vi "Automatic CE-CERT Inverter MODBUS TCP-IP Curtailment v2.vi"() -> ()   [LabVIEW 2018]
uses:
  <vilib>/Plasmionique/MB Master/MB_Master_TCP/MB_Master_TCP.lvclass
  C:/Program Files (x86)/National Instruments/LabVIEW 2018/vi.lib/Plasmionique/MB Master/MB_Master/MB_Master.lvclass
  <vilib>/Plasmionique/MB Master/MB Master.lvlib
panel:
  out "Current State Curtailment":T1(ring)
  in  "Curtailment Setpoint (%)":u16
  in  "Curtailment":bool
  in  "Power Factor":bool
  out "Inverter ready for commands?":bool
  in  "Power Factor Setpoint":i16
  out "Curtailment mode (should be 0 while not curtailing)":u16
  out "Power Factor Mode (should be 0 while not changing power factor)":u16
  out "Power Factor Operation Error (Should be 0)":u16
  out "Power Factor Format Error (Should be 0)":u16
  out "Current State Power Factor":T2(ring)
  in  "stop":bool
  in  "IP Address":string
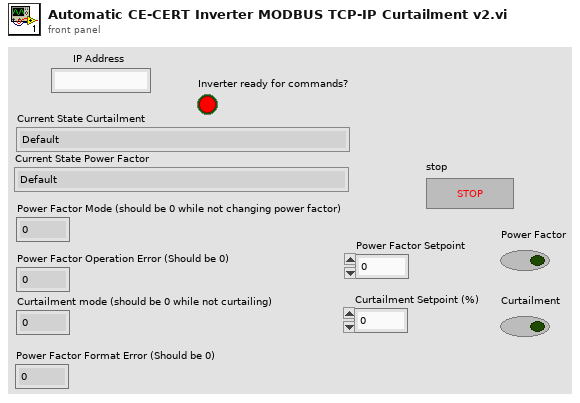
[diagram p1: front panel]
types:
  T1 = enum16{"Default", "Set advanced power control", "Set power factor mode", "set curtailment mode", "set ramp rate", "set action delay", "set randomize range", "set curtailment setpoint", "set go now command"}
  T2 = enum16{"Default", "Set Advanced power controls", "Set power factor mode", "set curtailment mode", "set action delay", "set ramp rate", "set randomize range", "set power factor setpoint", "set go now command"}
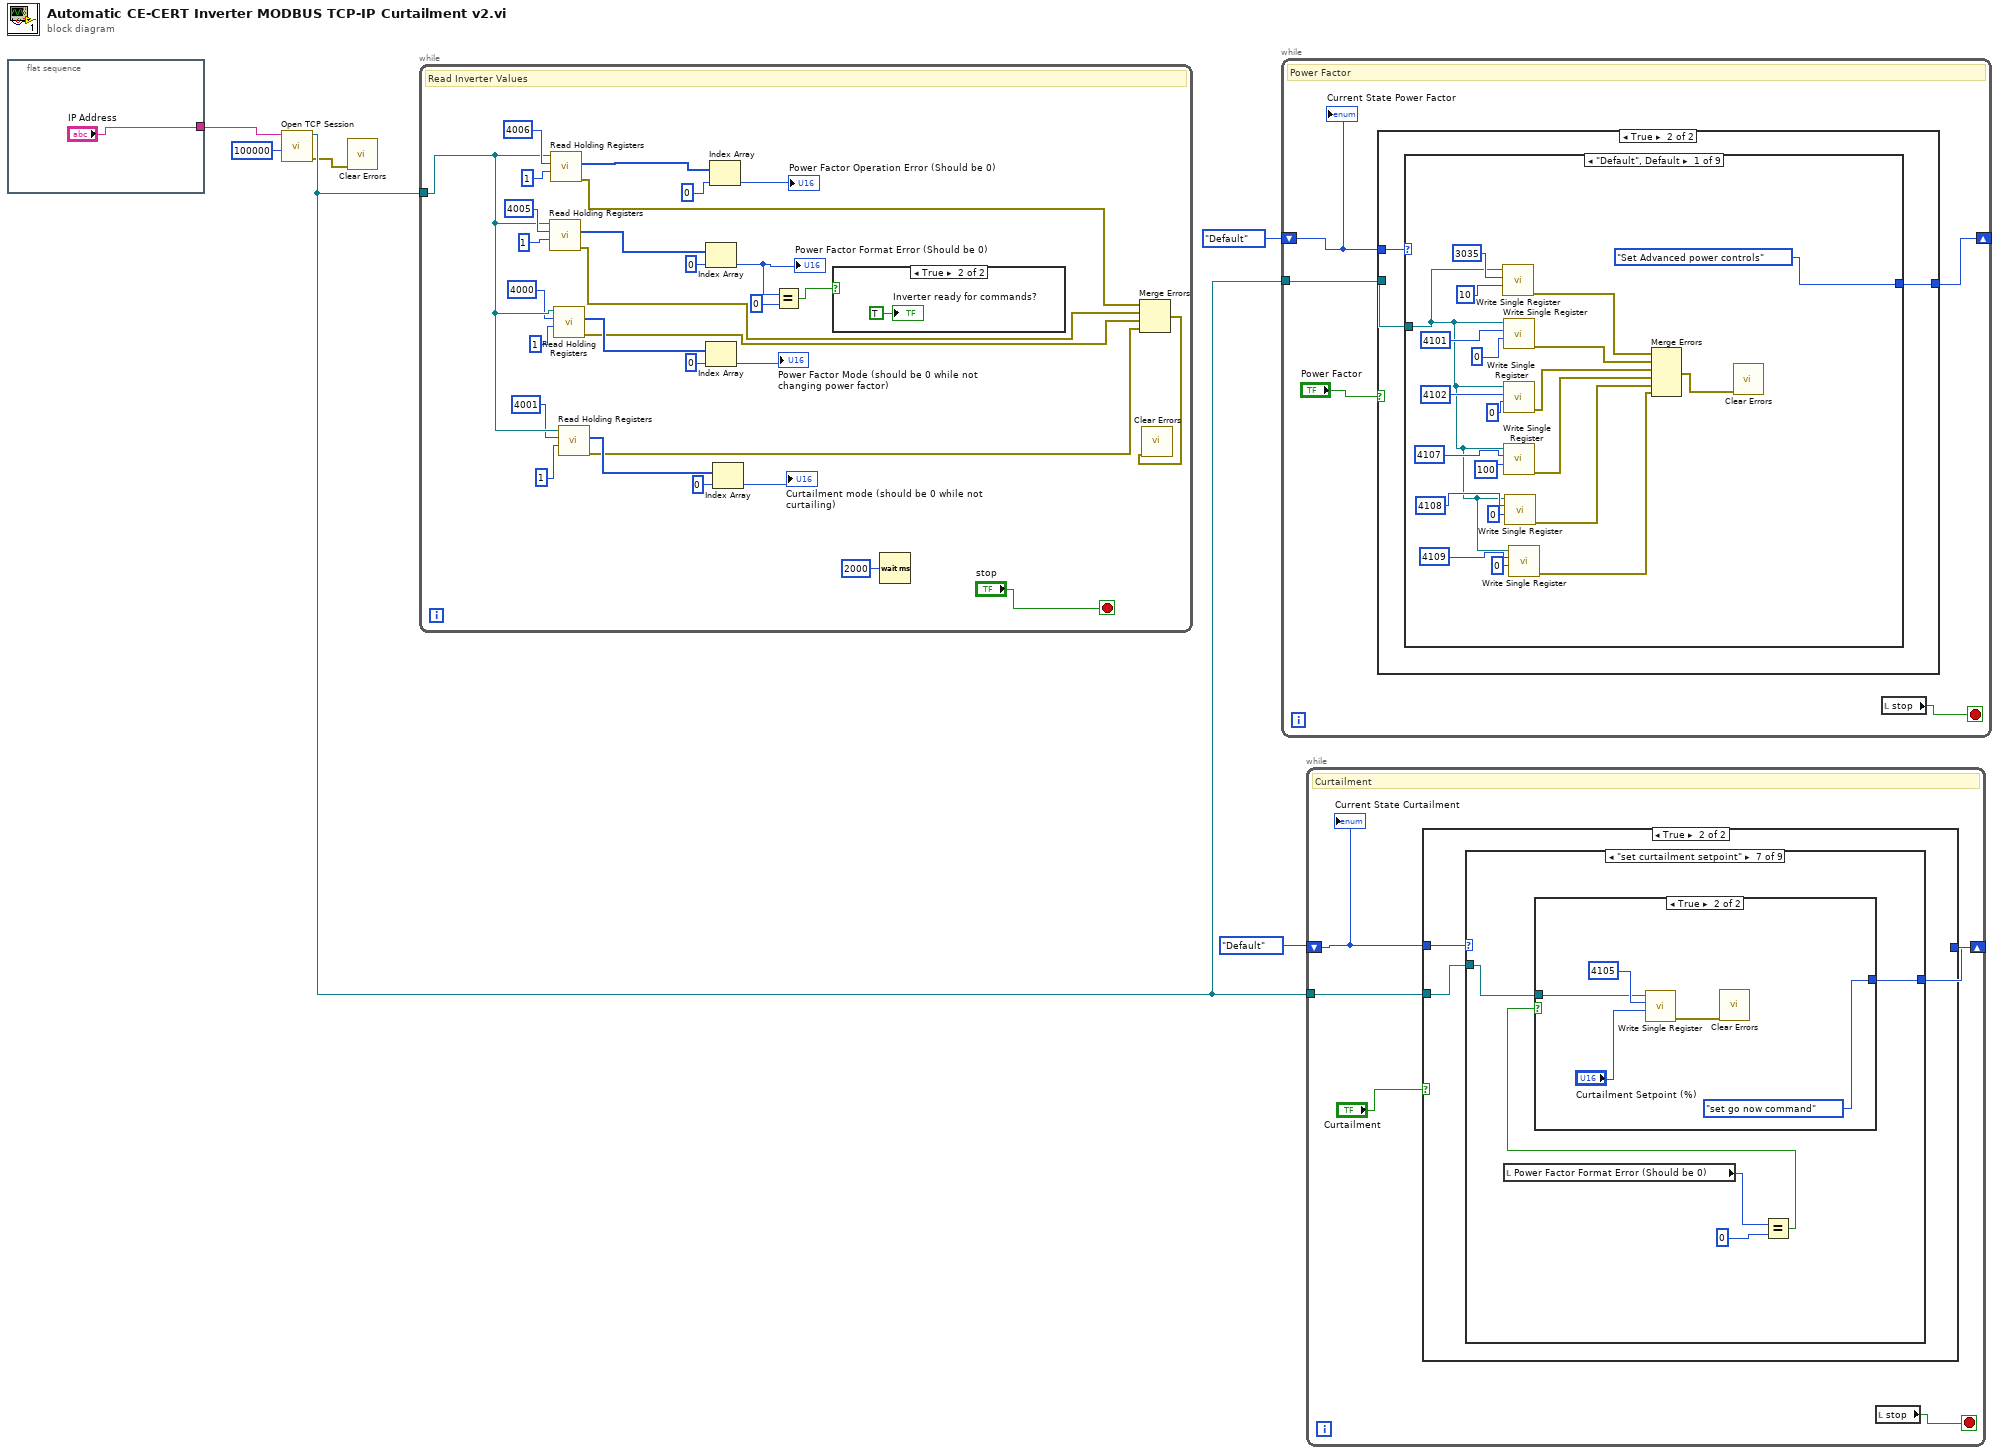
[diagram p0: block diagram]
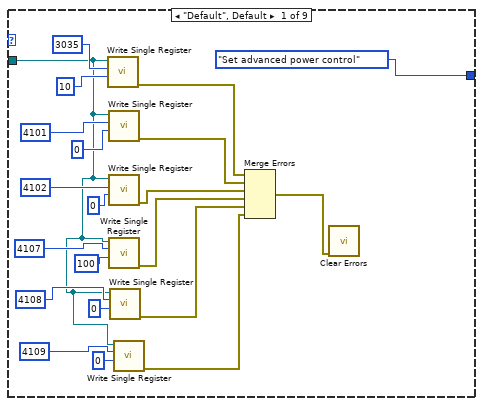
[diagram p3: hidden frame]
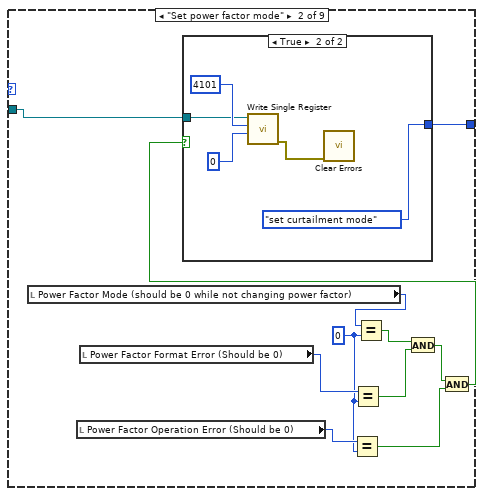
[diagram p4: hidden frame]
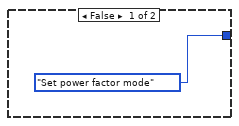
[diagram p5: hidden frame]
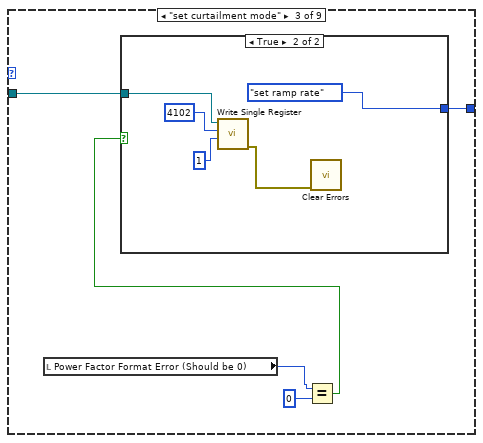
[diagram p6: hidden frame]
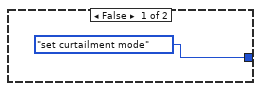
[diagram p7: hidden frame]
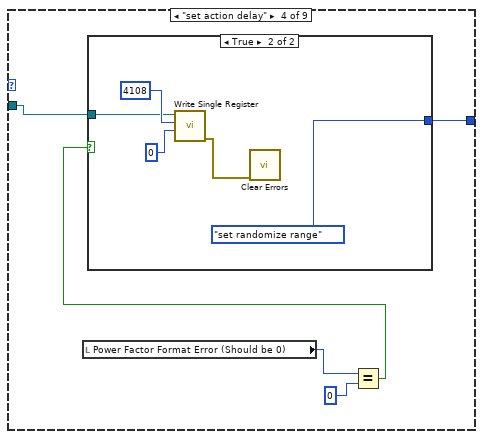
[diagram p8: hidden frame]
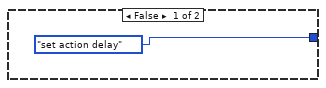
[diagram p9: hidden frame]
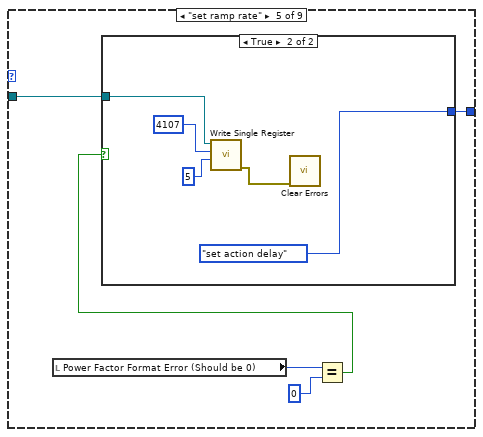
[diagram p10: hidden frame]
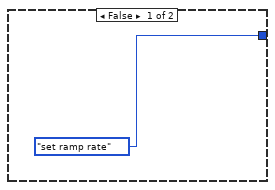
[diagram p11: hidden frame]
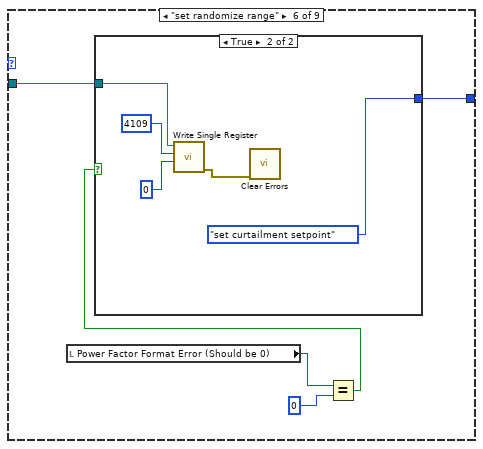
[diagram p12: hidden frame]
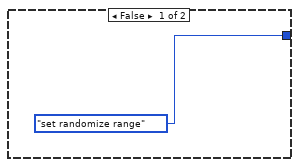
[diagram p13: hidden frame]
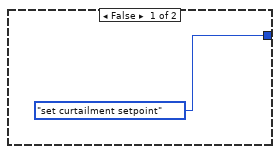
[diagram p14: hidden frame]
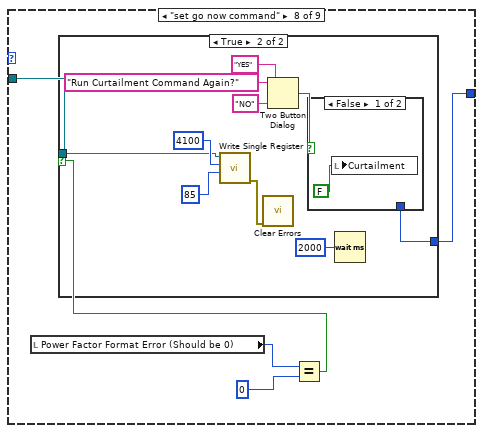
[diagram p15: hidden frame]
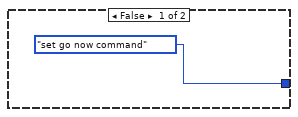
[diagram p16: hidden frame]
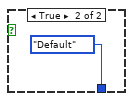
[diagram p17: hidden frame]
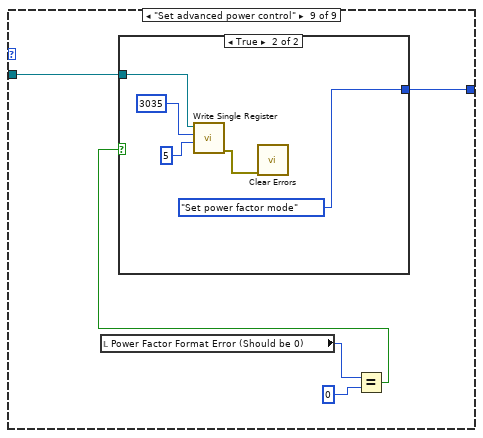
[diagram p18: hidden frame]
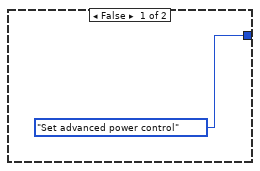
[diagram p19: hidden frame]
diagram:
  n1 = flat-sequence {
    tunnel: ["IP Address"] -> w6
    frame #0 {
    }
  }
  n2 = call <vilib>:"Open TCP Session.vi"("Timeout (10000)"=100000, "IP Address"=w6) -> ("error out"=w1:errorcluster, "MB_TCP session"=w3:refnum<class "MB_Master_TCP.lvclass">)  [unwired: 8 in]
  n3 = call <vilib>:"Clear Errors.vi"("error in (no error)"=w1) -> ()  [unwired: 5 in, 2 out]
  n4 = while {
    tunnel: w3 -> [w33]
    stop <- "stop" stop-if-true
    # "Read Inverter Values"
    n5 = call <vilib>:"Read Holding Registers.vi"("quantity"=u16 1, "starting address"=u16 4005, "MB session in"=w33) -> ("error out"=w11:errorcluster, "Registers"=w27:u16[])  [unwired: 6 in, 1 out]
    n6 = call <vilib>:"Read Holding Registers.vi"("quantity"=u16 1, "starting address"=u16 4006, "MB session in"=w33) -> ("error out"=w12:errorcluster, "Registers"=w25:u16[])  [unwired: 6 in, 1 out]
    n7 = call <vilib>:"Read Holding Registers.vi"("quantity"=u16 1, "starting address"=u16 4000, "MB session in"=w33) -> ("error out"=w10:errorcluster, "Registers"=w22:u16[])  [unwired: 6 in, 1 out]
    n8 = call <vilib>:"Read Holding Registers.vi"("quantity"=u16 1, "starting address"=u16 4001, "MB session in"=w33) -> ("error out"=w9:errorcluster, "Registers"=w19:u16[])  [unwired: 6 in, 1 out]
    n9 = Index Array(array=w27, index=0) -> (element=w16:u16)
    "Power Factor Format Error (Should be 0)" <- w16
    n10 = Index Array(array=w22, index=0) -> (element=→"Power Factor Mode (should be 0 while not changing power factor)":u16)
    n11 = Index Array(array=w25, index=0) -> (element=→"Power Factor Operation Error (Should be 0)":u16)
    n12 = Index Array(array=w19, index=0) -> (element=→"Curtailment mode (should be 0 while not curtailing)":u16)
    n13 = Equal?(x=w16, y=u16 0) -> (x = y?=w14:bool)
    n14 = case shown="True" w14 {
      frame False {
        n15 = local write "Inverter ready for commands?"(FALSE ("Inverter ready for commands")) -> ()
      }
      frame True {
        "Inverter ready for commands?" <- TRUE ("Inverter ready for commands")
      }
    }
    n16 = Wait (ms)(milliseconds to wait=u32 2000) -> ()  [unwired: 1 out]
    n17 = Merge Errors(w12, w11, w10, w9) -> (w8:errorcluster)
    n18 = call <vilib>:"Clear Errors.vi"("error in (no error)"=w8) -> ()  [unwired: 5 in, 2 out]
  }
  n19 = while {
    shift-right: [w41] -> _
    shift-left: T2."Default" -> [w43]
    tunnel: w3 -> [w42]
    stop <- w44 stop-if-true
    # "Power Factor"
    n20 = case shown="True" "Power Factor" {
      tunnel: w43 -> [_ w47]
      tunnel: w42 -> [_ w46]
      tunnel: [_ w45] -> w41
      frame False {
      }
      frame True {
        n21 = case shown="\"Default\", Default" w47 {
          tunnel: w46 -> [w56 w70 w87 w101 w109 w120 w131 w142 w160]
          tunnel: [T2."Set Advanced power controls" w69 w86 w97 w108 w119 w130 w141 w159] -> w45
          frame "Default", Default {
            n22 = call <vilib>:"Write Single Register.vi"("value"=u16 10, "address"=u16 3035, "MB session in"=w56) -> ("error out"=w54:errorcluster)  [unwired: 7 in, 1 out]
            n23 = call <vilib>:"Write Single Register.vi"("value"=u16 0, "address"=u16 4101, "MB session in"=w56) -> ("error out"=w53:errorcluster)  [unwired: 7 in, 1 out]
            n24 = call <vilib>:"Write Single Register.vi"("value"=u16 0, "address"=u16 4102, "MB session in"=w56) -> ("error out"=w52:errorcluster)  [unwired: 7 in, 1 out]
            n25 = call <vilib>:"Write Single Register.vi"("value"=u16 100, "address"=u16 4107, "MB session in"=w56) -> ("error out"=w51:errorcluster)  [unwired: 7 in, 1 out]
            n26 = call <vilib>:"Write Single Register.vi"("value"=u16 0, "address"=u16 4108, "MB session in"=w56) -> ("error out"=w50:errorcluster)  [unwired: 7 in, 1 out]
            n27 = call <vilib>:"Write Single Register.vi"("value"=u16 0, "address"=u16 4109, "MB session in"=w56) -> ("error out"=w49:errorcluster)  [unwired: 7 in, 1 out]
            n28 = Merge Errors(w54, w53, w52, w51, w50, w49) -> (w48:errorcluster)
            n29 = call <vilib>:"Clear Errors.vi"("error in (no error)"=w48) -> ()  [unwired: 5 in, 2 out]
          }
          frame "Set power factor mode" {
            w76 = u16 0 ("y")
            n30 = local read "Power Factor Mode (should be 0 while not changing power factor)"() -> (w79:u16)
            n31 = local read "Power Factor Operation Error (Should be 0)"() -> (w77:u16)
            n32 = local read "Power Factor Format Error (Should be 0)"() -> (w78:u16)
            n33 = Equal?(x=w77, y=w76) -> (x = y?=w72:bool)
            n34 = Equal?(x=w78, y=w76) -> (x = y?=w74:bool)
            n35 = Equal?(x=w79, y=w76) -> (x = y?=w75:bool)
            n36 = And(x=w75, y=w74) -> (x .and. y?=w73:bool)
            n37 = And(x=w73, y=w72) -> (x .and. y?=w71:bool)
            n38 = case shown="True" w71 {
              tunnel: w70 -> [_ w85]
              tunnel: [T2."Set power factor mode" T2."set curtailment mode"] -> w69
              frame False {
              }
              frame True {
                n39 = call <vilib>:"Write Single Register.vi"("value"=u16 1, "address"=u16 4101, "MB session in"=w85) -> ("error out"=w81:errorcluster)  [unwired: 7 in, 1 out]
                n40 = call <vilib>:"Clear Errors.vi"("error in (no error)"=w81) -> ()  [unwired: 5 in, 2 out]
              }
            }
          }
          frame "set curtailment mode" {
            n41 = local read "Power Factor Format Error (Should be 0)"() -> (w90:u16)
            n42 = Equal?(x=w90, y=u16 0) -> (x = y?=w88:bool)
            n43 = case shown="True" w88 {
              tunnel: w87 -> [_ w96]
              tunnel: [T2."set curtailment mode" T2."set action delay"] -> w86
              frame False {
              }
              frame True {
                n44 = call <vilib>:"Write Single Register.vi"("value"=u16 0, "address"=u16 4102, "MB session in"=w96) -> ("error out"=w92:errorcluster)  [unwired: 7 in, 1 out]
                n45 = call <vilib>:"Clear Errors.vi"("error in (no error)"=w92) -> ()  [unwired: 5 in, 2 out]
              }
            }
          }
          frame "set action delay" {
            n46 = local read "Power Factor Format Error (Should be 0)"() -> (w100:u16)
            n47 = Equal?(x=w100, y=u16 0) -> (x = y?=w98:bool)
            n48 = case shown="True" w98 {
              tunnel: w101 -> [_ w107]
              tunnel: [T2."set action delay" T2."set ramp rate"] -> w97
              frame False {
              }
              frame True {
                n49 = call <vilib>:"Write Single Register.vi"("value"=u16 0, "address"=u16 4108, "MB session in"=w107) -> ("error out"=w103:errorcluster)  [unwired: 7 in, 1 out]
                n50 = call <vilib>:"Clear Errors.vi"("error in (no error)"=w103) -> ()  [unwired: 5 in, 2 out]
              }
            }
          }
          frame "set ramp rate" {
            n51 = local read "Power Factor Format Error (Should be 0)"() -> (w111:u16)
            n52 = Equal?(x=w111, y=u16 0) -> (x = y?=w112:bool)
            n53 = case shown="True" w112 {
              tunnel: w109 -> [_ w118]
              tunnel: [T2."set ramp rate" T2."set randomize range"] -> w108
              frame False {
              }
              frame True {
                n54 = call <vilib>:"Write Single Register.vi"("value"=u16 100, "address"=u16 4107, "MB session in"=w118) -> ("error out"=w114:errorcluster)  [unwired: 7 in, 1 out]
                n55 = call <vilib>:"Clear Errors.vi"("error in (no error)"=w114) -> ()  [unwired: 5 in, 2 out]
              }
            }
          }
          frame "set randomize range" {
            n56 = local read "Power Factor Format Error (Should be 0)"() -> (w123:u16)
            n57 = Equal?(x=w123, y=u16 0) -> (x = y?=w121:bool)
            n58 = case shown="True" w121 {
              tunnel: w120 -> [_ w129]
              tunnel: [T2."set randomize range" T2."set power factor setpoint"] -> w119
              frame False {
              }
              frame True {
                n59 = call <vilib>:"Write Single Register.vi"("value"=u16 0, "address"=u16 4109, "MB session in"=w129) -> ("error out"=w125:errorcluster)  [unwired: 7 in, 1 out]
                n60 = call <vilib>:"Clear Errors.vi"("error in (no error)"=w125) -> ()  [unwired: 5 in, 2 out]
              }
            }
          }
          frame "set power factor setpoint" {
            n61 = local read "Power Factor Format Error (Should be 0)"() -> (w134:u16)
            n62 = Equal?(x=w134, y=u16 0) -> (x = y?=w132:bool)
            n63 = case shown="True" w132 {
              tunnel: w131 -> [_ w140]
              tunnel: [T2."set power factor setpoint" T2."set go now command"] -> w130
              frame False {
              }
              frame True {
                n64 = call <vilib>:"Write Single Register.vi"("value"="Power Factor Setpoint", "address"=u16 4103, "MB session in"=w140) -> ("error out"=w136:errorcluster)  [unwired: 7 in, 1 out]
                n65 = call <vilib>:"Clear Errors.vi"("error in (no error)"=w136) -> ()  [unwired: 5 in, 2 out]
              }
            }
          }
          frame "set go now command" {
            n66 = local read "Power Factor Format Error (Should be 0)"() -> (w145:u16)
            n67 = Equal?(x=w145, y=u16 0) -> (x = y?=w143:bool)
            n68 = case shown="True" w143 {
              tunnel: w142 -> [_ w156]
              tunnel: [T2."set go now command" w153] -> w141
              frame False {
              }
              frame True {
                n69 = call <vilib>:"Write Single Register.vi"("value"=u16 85, "address"=u16 4100, "MB session in"=w156) -> ("error out"=w147:errorcluster)  [unwired: 7 in, 1 out]
                n70 = Two Button Dialog(message="Run Power Factor Command again?", 1:"NO" ("T button name (\"OK\")"), 2:"YES" ("T button name (\"OK\")")) -> (T button?=w151:bool)
                n71 = call <vilib>:"Clear Errors.vi"("error in (no error)"=w147) -> ()  [unwired: 5 in, 2 out]
                n72 = case shown="True" w151 {
                  tunnel: [_ T2."Default"] -> w153
                  frame False {
                    n73 = local write "Power Factor"(FALSE ("Power Factor")) -> ()
                  }
                  frame True {
                  }
                }
                n74 = Wait (ms)(milliseconds to wait=u32 2000) -> ()  [unwired: 1 out]
              }
            }
          }
          frame "Set Advanced power controls" {
            n75 = local read "Power Factor Format Error (Should be 0)"() -> (w163:u16)
            n76 = Equal?(x=w163, y=u16 0) -> (x = y?=w161:bool)
            n77 = case shown="True" w161 {
              tunnel: w160 -> [_ w169]
              tunnel: [T2."Set Advanced power controls" T2."Set power factor mode"] -> w159
              frame False {
              }
              frame True {
                n78 = call <vilib>:"Write Single Register.vi"("value"=u16 5, "address"=u16 3035, "MB session in"=w169) -> ("error out"=w165:errorcluster)  [unwired: 7 in, 1 out]
                n79 = call <vilib>:"Clear Errors.vi"("error in (no error)"=w165) -> ()  [unwired: 5 in, 2 out]
              }
            }
          }
        }
      }
    }
    n80 = local read "stop"() -> (w44:bool)
    "Current State Power Factor" <- w43
  }
  n81 = while {
    tunnel: w3 -> [w173]
    shift-right: [w172] -> _
    shift-left: T1."Default" -> [w171]
    stop <- w174 stop-if-true
    # "Curtailment"
    n82 = case shown="True" "Curtailment" {
      tunnel: w173 -> [_ w177]
      tunnel: [_ w176] -> w172
      tunnel: w171 -> [_ w175]
      frame False {
      }
      frame True {
        n83 = case shown="\"set curtailment setpoint\"" w175 {
          tunnel: w177 -> [w186 w199 w216 w227 w238 w249 w260 w271 w289]
          tunnel: [T1."Set advanced power control" w200 w217 w228 w239 w250 w261 w272 w290] -> w176
          frame "Default", Default {
            n84 = call <vilib>:"Write Single Register.vi"("value"=u16 10, "address"=u16 3035, "MB session in"=w186) -> ("error out"=w184:errorcluster)  [unwired: 7 in, 1 out]
            n85 = call <vilib>:"Write Single Register.vi"("value"=u16 0, "address"=u16 4101, "MB session in"=w186) -> ("error out"=w183:errorcluster)  [unwired: 7 in, 1 out]
            n86 = call <vilib>:"Write Single Register.vi"("value"=u16 0, "address"=u16 4102, "MB session in"=w186) -> ("error out"=w182:errorcluster)  [unwired: 7 in, 1 out]
            n87 = call <vilib>:"Write Single Register.vi"("value"=u16 100, "address"=u16 4107, "MB session in"=w186) -> ("error out"=w181:errorcluster)  [unwired: 7 in, 1 out]
            n88 = call <vilib>:"Write Single Register.vi"("value"=u16 0, "address"=u16 4108, "MB session in"=w186) -> ("error out"=w180:errorcluster)  [unwired: 7 in, 1 out]
            n89 = call <vilib>:"Write Single Register.vi"("value"=u16 0, "address"=u16 4109, "MB session in"=w186) -> ("error out"=w179:errorcluster)  [unwired: 7 in, 1 out]
            n90 = Merge Errors(w184, w183, w182, w181, w180, w179) -> (w178:errorcluster)
            n91 = call <vilib>:"Clear Errors.vi"("error in (no error)"=w178) -> ()  [unwired: 5 in, 2 out]
          }
          frame "Set power factor mode" {
            w206 = u16 0 ("y")
            n92 = local read "Power Factor Mode (should be 0 while not changing power factor)"() -> (w209:u16)
            n93 = local read "Power Factor Operation Error (Should be 0)"() -> (w207:u16)
            n94 = local read "Power Factor Format Error (Should be 0)"() -> (w208:u16)
            n95 = Equal?(x=w207, y=w206) -> (x = y?=w202:bool)
            n96 = Equal?(x=w208, y=w206) -> (x = y?=w204:bool)
            n97 = Equal?(x=w209, y=w206) -> (x = y?=w205:bool)
            n98 = And(x=w205, y=w204) -> (x .and. y?=w203:bool)
            n99 = And(x=w203, y=w202) -> (x .and. y?=w201:bool)
            n100 = case shown="True" w201 {
              tunnel: [T1."Set power factor mode" T1."set curtailment mode"] -> w200
              tunnel: w199 -> [_ w212]
              frame False {
              }
              frame True {
                n101 = call <vilib>:"Write Single Register.vi"("value"=u16 0, "address"=u16 4101, "MB session in"=w212) -> ("error out"=w211:errorcluster)  [unwired: 7 in, 1 out]
                n102 = call <vilib>:"Clear Errors.vi"("error in (no error)"=w211) -> ()  [unwired: 5 in, 2 out]
              }
            }
          }
          frame "set curtailment mode" {
            n103 = local read "Power Factor Format Error (Should be 0)"() -> (w220:u16)
            n104 = Equal?(x=w220, y=u16 0) -> (x = y?=w218:bool)
            n105 = case shown="True" w218 {
              tunnel: [T1."set curtailment mode" T1."set ramp rate"] -> w217
              tunnel: w216 -> [_ w223]
              frame False {
              }
              frame True {
                n106 = call <vilib>:"Write Single Register.vi"("value"=u16 1, "address"=u16 4102, "MB session in"=w223) -> ("error out"=w222:errorcluster)  [unwired: 7 in, 1 out]
                n107 = call <vilib>:"Clear Errors.vi"("error in (no error)"=w222) -> ()  [unwired: 5 in, 2 out]
              }
            }
          }
          frame "set action delay" {
            n108 = local read "Power Factor Format Error (Should be 0)"() -> (w231:u16)
            n109 = Equal?(x=w231, y=u16 0) -> (x = y?=w229:bool)
            n110 = case shown="True" w229 {
              tunnel: [T1."set action delay" T1."set randomize range"] -> w228
              tunnel: w227 -> [_ w234]
              frame False {
              }
              frame True {
                n111 = call <vilib>:"Write Single Register.vi"("value"=u16 0, "address"=u16 4108, "MB session in"=w234) -> ("error out"=w233:errorcluster)  [unwired: 7 in, 1 out]
                n112 = call <vilib>:"Clear Errors.vi"("error in (no error)"=w233) -> ()  [unwired: 5 in, 2 out]
              }
            }
          }
          frame "set ramp rate" {
            n113 = local read "Power Factor Format Error (Should be 0)"() -> (w241:u16)
            n114 = Equal?(x=w241, y=u16 0) -> (x = y?=w242:bool)
            n115 = case shown="True" w242 {
              tunnel: [T1."set ramp rate" T1."set action delay"] -> w239
              tunnel: w238 -> [_ w245]
              frame False {
              }
              frame True {
                n116 = call <vilib>:"Write Single Register.vi"("value"=u16 5, "address"=u16 4107, "MB session in"=w245) -> ("error out"=w244:errorcluster)  [unwired: 7 in, 1 out]
                n117 = call <vilib>:"Clear Errors.vi"("error in (no error)"=w244) -> ()  [unwired: 5 in, 2 out]
              }
            }
          }
          frame "set randomize range" {
            n118 = local read "Power Factor Format Error (Should be 0)"() -> (w253:u16)
            n119 = Equal?(x=w253, y=u16 0) -> (x = y?=w251:bool)
            n120 = case shown="True" w251 {
              tunnel: [T1."set randomize range" T1."set curtailment setpoint"] -> w250
              tunnel: w249 -> [_ w256]
              frame False {
              }
              frame True {
                n121 = call <vilib>:"Write Single Register.vi"("value"=u16 0, "address"=u16 4109, "MB session in"=w256) -> ("error out"=w255:errorcluster)  [unwired: 7 in, 1 out]
                n122 = call <vilib>:"Clear Errors.vi"("error in (no error)"=w255) -> ()  [unwired: 5 in, 2 out]
              }
            }
          }
          frame "set curtailment setpoint" {
            n123 = local read "Power Factor Format Error (Should be 0)"() -> (w264:u16)
            n124 = Equal?(x=w264, y=u16 0) -> (x = y?=w262:bool)
            n125 = case shown="True" w262 {
              tunnel: [T1."set curtailment setpoint" T1."set go now command"] -> w261
              tunnel: w260 -> [_ w267]
              frame False {
              }
              frame True {
                n126 = call <vilib>:"Write Single Register.vi"("value"="Curtailment Setpoint (%)", "address"=u16 4105, "MB session in"=w267) -> ("error out"=w266:errorcluster)  [unwired: 7 in, 1 out]
                n127 = call <vilib>:"Clear Errors.vi"("error in (no error)"=w266) -> ()  [unwired: 5 in, 2 out]
              }
            }
          }
          frame "set go now command" {
            n128 = local read "Power Factor Format Error (Should be 0)"() -> (w275:u16)
            n129 = Equal?(x=w275, y=u16 0) -> (x = y?=w273:bool)
            n130 = case shown="True" w273 {
              tunnel: [T1."set go now command" w279] -> w272
              tunnel: w271 -> [_ w284]
              frame False {
              }
              frame True {
                n131 = call <vilib>:"Write Single Register.vi"("value"=u16 85, "address"=u16 4100, "MB session in"=w284) -> ("error out"=w277:errorcluster)  [unwired: 7 in, 1 out]
                n132 = call <vilib>:"Clear Errors.vi"("error in (no error)"=w277) -> ()  [unwired: 5 in, 2 out]
                n133 = Two Button Dialog(message="Run Curtailment Command Again?", 1:"NO" ("F button name (\"Cancel\")"), 2:"YES" ("T button name (\"OK\")")) -> (T button?=w283:bool)
                n134 = case shown="False" w283 {
                  tunnel: [_ T1."Default"] -> w279
                  frame False {
                    n135 = local write "Curtailment"(FALSE ("Curtailment")) -> ()
                  }
                  frame True {
                  }
                }
                n136 = Wait (ms)(milliseconds to wait=u32 2000) -> ()  [unwired: 1 out]
              }
            }
          }
          frame "Set advanced power control" {
            n137 = local read "Power Factor Format Error (Should be 0)"() -> (w293:u16)
            n138 = Equal?(x=w293, y=u16 0) -> (x = y?=w291:bool)
            n139 = case shown="True" w291 {
              tunnel: [T1."Set advanced power control" T1."Set power factor mode"] -> w290
              tunnel: w289 -> [_ w296]
              frame False {
              }
              frame True {
                n140 = call <vilib>:"Write Single Register.vi"("value"=u16 5, "address"=u16 3035, "MB session in"=w296) -> ("error out"=w295:errorcluster)  [unwired: 7 in, 1 out]
                n141 = call <vilib>:"Clear Errors.vi"("error in (no error)"=w295) -> ()  [unwired: 5 in, 2 out]
              }
            }
          }
        }
      }
    }
    n142 = local read "stop"() -> (w174:bool)
    "Current State Curtailment" <- w171
  }
